vi "Read DriveForward.vi"(8 "error in (no error)":errorcluster, 11 "DriverXBoxController in":refnum<class "DriverXBoxController.lvclass">) -> (0 "error out":errorcluster, 2 "Forward":dbl(slide) scale=-1.0..1.0, 3 "DriverXBoxController out":refnum<class "DriverXBoxController.lvclass">)   [LabVIEW 2013, in "DriverXBoxController.lvclass"]
uses:
  DriverXBoxController.lvclass
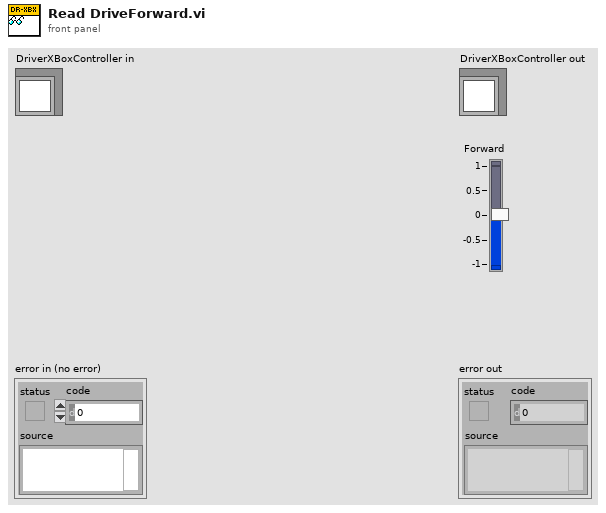
[diagram p1: front panel]
types:
  T1 = cluster{"LeftJoystick":cluster{"Forward":dbl, "Right":dbl}, "RightJoystick":cluster{"Forward":dbl, "Right":dbl}}
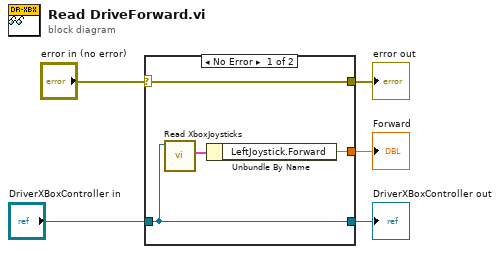
[diagram p0: block diagram]
diagram:
  n1 = case shown="No Error" "error in (no error)" {
    selector: "error in (no error)" -> [w9 w10]
    tunnel: [w9 w10] -> w4
    tunnel: [w8 w11] -> w2
    tunnel: "DriverXBoxController in" -> [w8 w11]
    tunnel: [w6 _] -> w1
    frame No Error {
      n2 = call-dynamic "Read XboxJoysticks.vi"("XBoxController in"=w8) -> ("XboxJoysticks"=w7:T1)  [unwired: 8 in, 2 out]
      n3 = Unbundle By Name(w7) -> ("LeftJoystick.Forward"=w6:dbl)
    }
    frame Error {
    }
  }
  "error out" <- w4
  "DriverXBoxController out" <- w2
  "Forward" <- w1
